vi "Generic Plugin UI.vi"() -> ()   [LabVIEW 2011, in "Generic Plugin.lvclass"]
uses:
  Generic Plugin.lvclass
panel:
  in  "Boolean":bool
  # "NO PLUGIN UI HAS BEEN DEFINED FOR THIS ITEM"
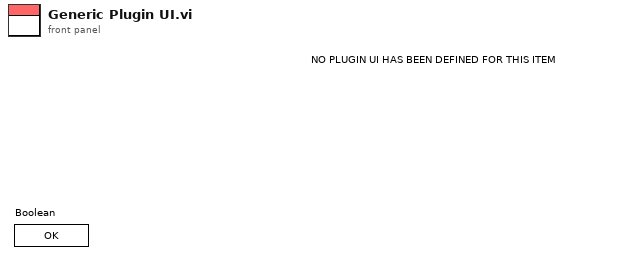
[diagram p1: front panel]
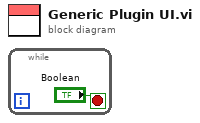
[diagram p0: block diagram]
diagram:
  n1 = while {
    stop <- "Boolean" stop-if-true
  }
